vi "I2C_Host_Read_2.vi"(8 "error in":errorcluster, 9 "IRQ Number":i32, 10 "NumBytesToRead":i32, 11 "FPGA VI Reference In":T1) -> (0 "error out":errorcluster, 1 "Status":i16, 2 "DataBytes":u8[](array[numeric]) caption="Data Byte" format="%.0x", 3 "FPGA VI Reference Out":T1)   [LabVIEW 2019]
doc: "Waits for the IRQ to be set by the FPGA that signifies the Data bytes requested are in the 'READ' memory block. Once this IRQ is received the data is read from the 'READ' memory block. The data bytes are read in one byte at a time using a for loop.\n\nNote: On recompiles the 'FPGA VI Reference' control may need to be updated. \nC:\\I2C_Core\\Controls\\FPGA_Reference.ctl\n\nVI Written By:\nPeter Fuller\nSenior Engineer\nplf Consulting, LLC"
uses:
  <vilib>/rvi/interface/nirviReadWriteControl/nirviReadWriteControl.xnode
  Controls/FPGA_Reference.ctl
  FPGA Bitfiles/LS_Durability_FPGA_9627.lvbitx
  <vilib>/rvi/errors/niLvFpgaMergeErrorWithErrorCode.vi
  <vilib>/rvi/errors/niLvFpgaAdjustHostInterfaceError.vi
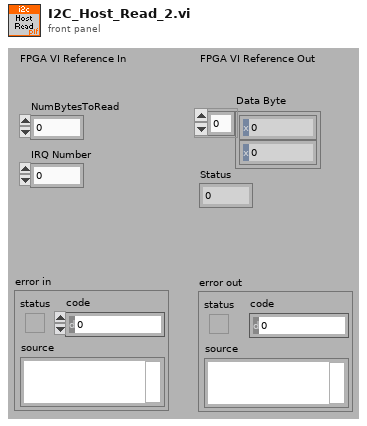
[diagram p1: front panel]
types:
  T1 = typedef "FPGA_Reference.ctl" = refnum<k20>
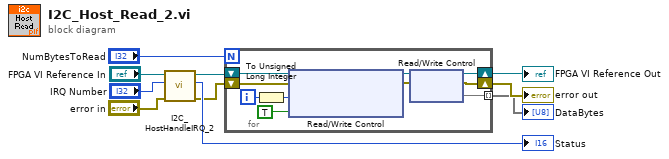
[diagram p0: block diagram]
diagram:
  n1 = call "I2C_HostHandleIRQ_2.vi"("error in"="error in", "IRQ Number"="IRQ Number", "FPGA VI Reference In"="FPGA VI Reference In") -> ("error out"=w1:errorcluster, "Status"=→"Status":i16, "FPGA VI Reference Out"=w2:T1)  [unwired: 6 in]
  n2 = for {
    N: "NumBytesToRead" -> [_]
    shift-right: [w13] -> w10
    shift-left: w2 -> [w20]
    shift-right: [w12] -> w9
    shift-left: w1 -> [w19]
    tunnel: [w11] -> w8 mode=indexing
    i -> [w18]
    n3 = To Unsigned Long Integer(number=w18) -> (unsigned 32bit integer=w17:u32)
    n4 = xnode "Read/Write Control"("FPGA VI Reference In"=w20, "error in"=w19, "MemoryAddress 2"=w17, "GetRead 2"=TRUE ("UpdateWrite")) -> ("FPGA VI Reference Out"=w15:T1, "error out"=w14:errorcluster)
    n5 = xnode "Read/Write Control"("FPGA VI Reference In"=w15, "error in"=w14) -> ("FPGA VI Reference Out"=w13:T1, "error out"=w12:errorcluster, "Data 2"=w11)
  }
  "DataBytes" <- w8
  "error out" <- w9
  "FPGA VI Reference Out" <- w10
